vi "Asynchronous Engine.vi"(8 "error in":errorcluster, 10 "Parent":string, 11 "Parameters":T1) -> ()   [LabVIEW 2015, in "Waveform-Processing-Custom-Device Engine.lvlib"]
uses:
  Waveform-Processing-Custom-Device Engine.lvlib
  Userlib/Error Handling API/Error Handling API.lvlib
  Shared/Running Average/Running Average.lvlib
  Userlib/Inline Async API/Inline Async API.lvlib
  Shared/Single-Point/SinglePoint.lvlib
  <vilib>/NI Veristand/Custom Device Tools/Custom Device Utility Library/Custom Device Utility Library.lvlib
  Types/Async FIFOs.ctl
  <vilib>/NI Veristand/Custom Device API/Waveform Data Reference.ctl
  <vilib>/NI VeriStand/Custom Device API/Custom Device API.lvlib
  Types/Async Parameters.ctl
panel:
  in  "Stop":bool
  out "error out":errorcluster
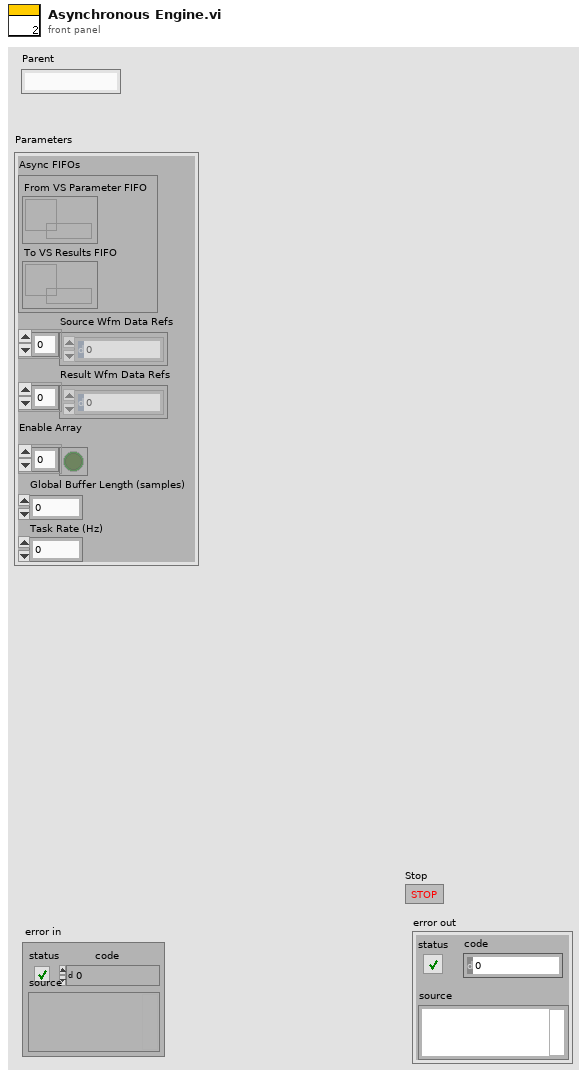
[diagram p1: front panel]
types:
  T1 = typedef "Waveform-Processing-Custom-Device Engine.lvlib/Async Parameters.ctl" = cluster{"Async FIFOs":T2, "Source Wfm Data Refs":T3[], "Result Wfm Data Refs":T3[], "Enable Array":bool[], "Global Buffer Length (samples)":dbl, "Task Rate (Hz)":dbl}
  T2 = typedef "Waveform-Processing-Custom-Device Engine.lvlib/Async FIFOs.ctl" = cluster{"From VS Parameter FIFO":refnum<k33>, "To VS Results FIFO":refnum<k33>}
  T3 = typedef "Custom Device API.lvlib/Waveform Data Reference.ctl" = i32
  T4 = typedef "Waveform-Processing-Custom-Device Engine.lvlib/Async State Vars.ctl" = cluster{"Async FIFOs":T2, "Source Wfm Session Refs":refnum<class "Single Waveform Read (DBL).lvclass">[], "Result Wfm Session Refs":refnum<class "Single Waveform Write (DBL).lvclass">[], "Result Wfm Data":dbl[][], "Source Wfm Data Refs":T3[], "Result Wfm Data Refs":T3[], "Global Buffer Length (samples)":dbl, "Parameter Array":dbl[], "Tag Results":dbl[], "Enable Array":bool[], "Task Rate":dbl}
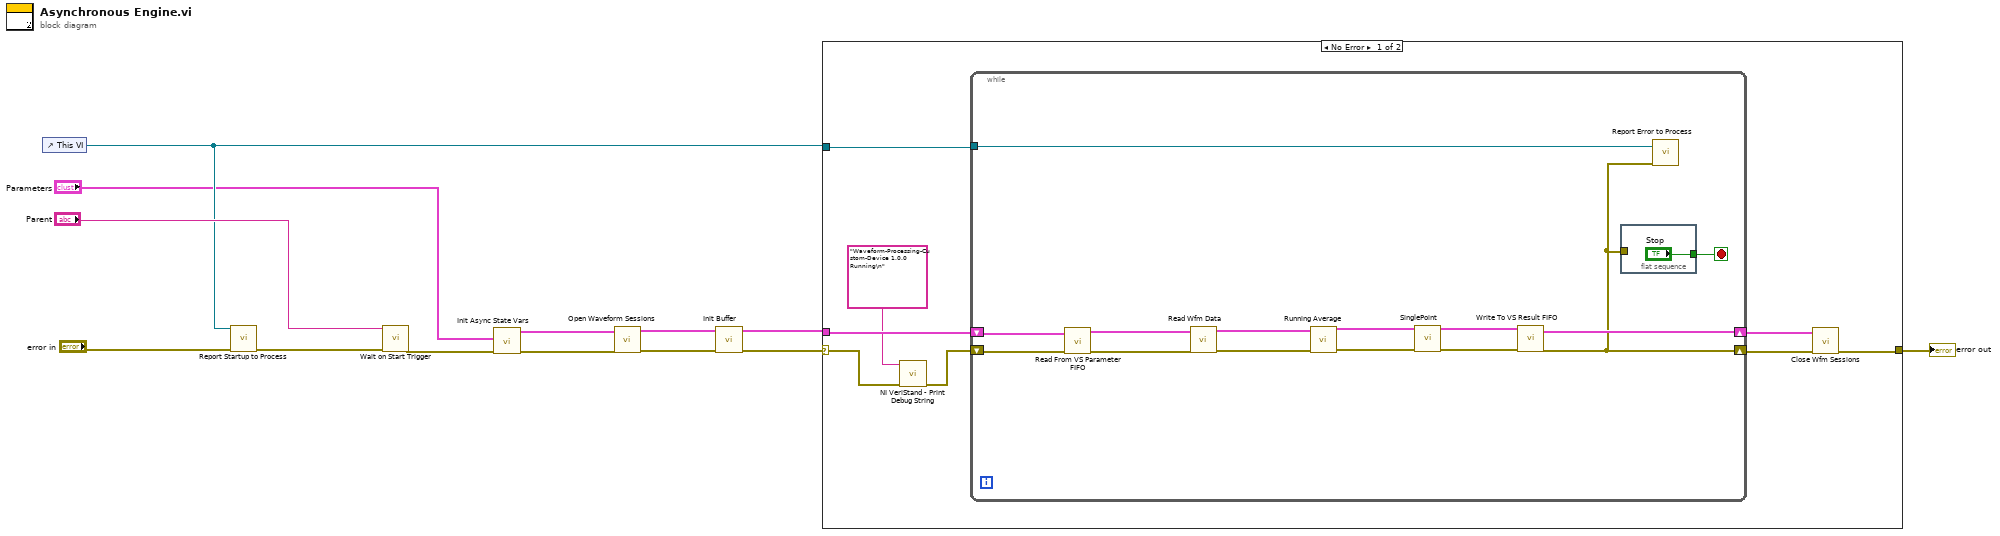
[diagram p0: block diagram]
diagram:
  n1 = control-ref of="This VI"() -> (w11:refnum<vi>)
  n2 = call "Report Startup to Process.vi"("Error"="error in", "This VI"=w11) -> ("error out"=w13:errorcluster)  [unwired: 9 in]
  n3 = call "Wait on Start Trigger.vi"("error in (no error)"=w13, "Name"="Parent") -> ("error out"=w10:errorcluster)  [unwired: 8 in, 1 out]
  n4 = call "Init Async State Vars.vi"("Error in"=w10, "Async Parameters"="Parameters") -> ("Error out"=w9:errorcluster, "Async State Vars"=w8:T4)  [unwired: 8 in]
  n5 = call "Open Waveform Sessions.vi"("error in"=w9, "Async State Vars"=w8) -> ("error out"=w5:errorcluster, "Async State Vars out"=w4:T4)  [unwired: 8 in]
  n6 = call "Init Buffer.vi"("Error in"=w5, "Async State Vars"=w4) -> ("Error out"=w6:errorcluster, "Async State Vars out"=w3:T4)  [unwired: 8 in]
  n7 = case shown="No Error" w6 {
    selector: w6 -> [w17 w37]
    tunnel: w11 -> [w21 _]
    tunnel: [w19 w37] -> w2
    tunnel: w3 -> [w15 _]
    frame No Error {
      n8 = call <vilib>:"NI VeriStand - Print Debug String.vi"("error in (no error)"=w17, "Message"="Waveform-Processing-Custom-Device 1.0.0 Running\n") -> ("error out"=w16:errorcluster)  [unwired: 9 in]
      n9 = while {
        shift-right: [w23] -> w20
        shift-left: w16 -> [w32]
        tunnel: w21 -> [w35]
        shift-right: [w28] -> w18
        shift-left: w15 -> [w33]
        stop <- w22 stop-if-true
        n10 = call "Read From VS Parameter FIFO.vi"("Error In"=w32, "Async State Vars"=w33) -> ("Error Out"=w31:errorcluster, "Async State Vars out"=w30:T4)  [unwired: 7 in, 1 out]
        n11 = call "Read Wfm Data.vi"("error in (no error)"=w31, "Async State Vars in"=w30) -> ("error out"=w34:errorcluster, "Async State Vars out"=w29:T4)  [unwired: 7 in, 1 out]
        n12 = call "Running Average.vi"("Error In"=w34, "Async State Vars 2"=w29) -> ("Error Out"=w27:errorcluster, "Async State Vars out"=w24:T4)  [unwired: 8 in]
        n13 = call "SinglePoint.vi"("Error In 2"=w27, "Async State Vars 2"=w24) -> ("Error Out"=w26:errorcluster, "Async State Vars out"=w25:T4)  [unwired: 8 in]
        n14 = call "Write To VS Result FIFO.vi"("Error in"=w26, "Async State Vars"=w25) -> ("Error out"=w23:errorcluster, "Async State Vars out"=w28:T4)  [unwired: 8 in]
        n15 = flat-sequence {
          tunnel: w23 -> [_]
          tunnel: ["Stop"] -> w22
          frame #0 {
          }
        }
        n16 = call "Report Error to Process.vi"("Error"=w23, "This VI"=w35) -> ()  [unwired: 10 in]
      }
      n17 = call "Close Wfm Sessions.vi"("Error In"=w20, "Async State Vars"=w18) -> ("Error Out"=w19:errorcluster)  [unwired: 9 in]
    }
    frame Error {
    }
  }
  "error out" <- w2
